vi "Untitled 1.vi"() -> ()   [LabVIEW 2020]
panel:
  in  "VISA resource name":refnum<visa-resource-name>
  in  "Table Control":string[][](table)
  out "Temp":dbl(graph)
  out "Thermometer":dbl(slide) scale=0.0..100.0
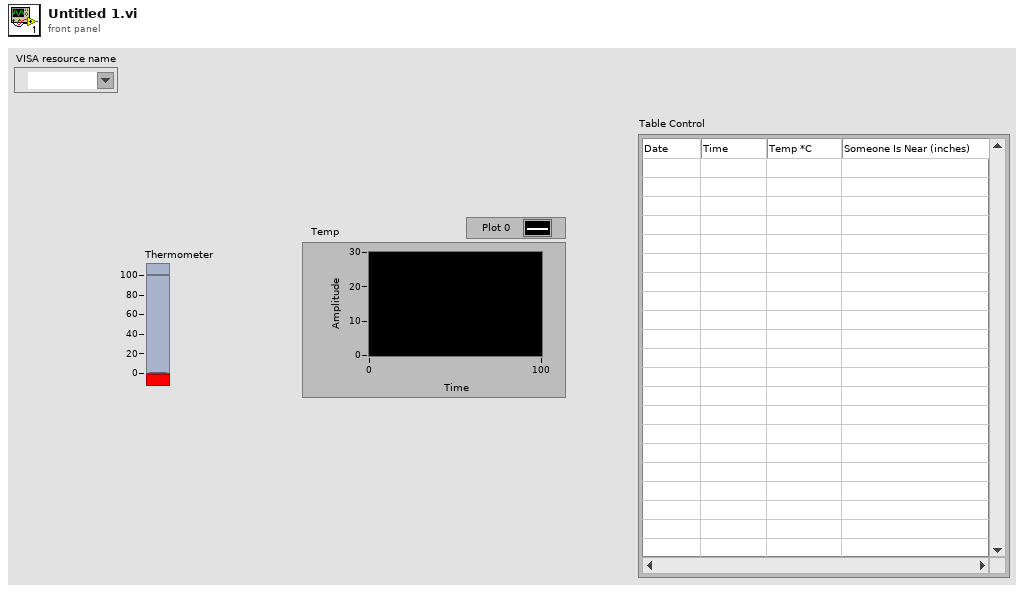
[diagram p1: front panel]
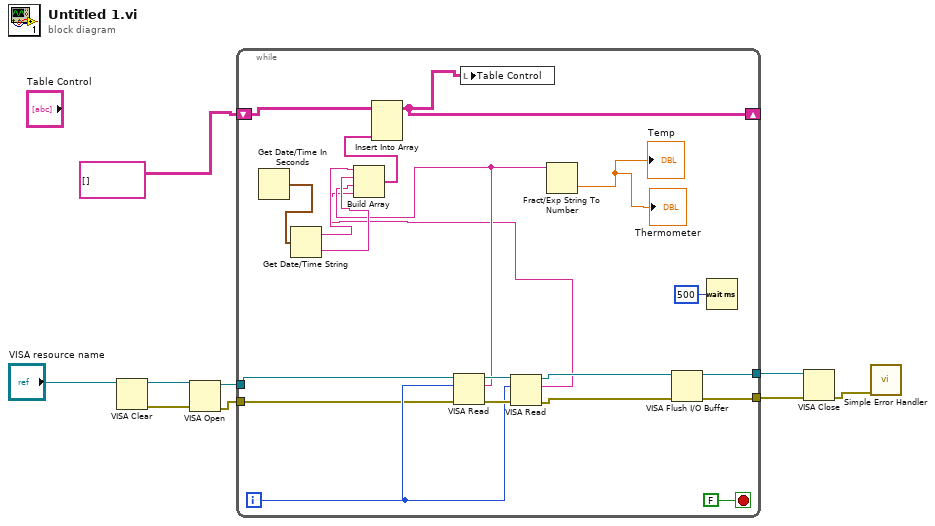
[diagram p0: block diagram]
diagram:
  n1 = VISA Clear(VISA resource name="VISA resource name") -> (VISA resource name out=w5:refnum<visa-resource-name>, error out=w6:errorcluster)  [unwired: 1 in]
  n2 = VISA Open(error in (no error)=w6, VISA resource name=w5) -> (VISA resource name=w4:refnum<visa-resource-name>, error out=w3:errorcluster)  [unwired: 3 in]
  n3 = while {
    tunnel: [w29] -> w8
    tunnel: [w28] -> w7
    tunnel: w4 -> [w22]
    tunnel: w3 -> [w21]
    shift-right: [w18] -> _
    shift-left: string[][] [] -> [w19]
    i -> [w23]
    stop <- FALSE stop-if-true
    n4 = Get Date/Time In Seconds() -> (seconds since 1Jan1904=w16:timestamp)
    n5 = Get Date/Time String(seconds (now)=w16) -> (date string=w15:string, time string=w14:string)  [unwired: 2 in]
    n6 = VISA Read(VISA resource name=w22, byte count=w23, error in (no error)=w21) -> (VISA resource name out=w25:refnum<visa-resource-name>, read buffer=w13:string, error out=w24:errorcluster)  [unwired: 1 out]
    n7 = VISA Read(VISA resource name=w25, byte count=w23, error in (no error)=w24) -> (VISA resource name out=w27:refnum<visa-resource-name>, read buffer=w11:string, error out=w26:errorcluster)  [unwired: 1 out]
    n8 = Build Array(w15, w14, w13, w11) -> (w10:string[])
    n9 = Insert Into Array(array=w19, new element=w10) -> (w18:string[][])  [unwired: 2 in]
    n10 = local write "Table Control"(w18) -> ()
    n11 = Fract/Exp String To Number(string=w13) -> (number=→"Thermometer" →"Temp":dbl)  [unwired: 3 in, 1 out]
    n12 = VISA Flush I/O Buffer(VISA resource name=w27, error in (no error)=w26) -> (VISA resource name out=w29:refnum<visa-resource-name>, error out=w28:errorcluster)  [unwired: 1 in]
    n13 = Wait (ms)(milliseconds to wait=u32 500) -> ()  [unwired: 1 out]
  }
  n14 = VISA Close(VISA resource name=w8, error in (no error)=w7) -> (error out=w9:errorcluster)
  n15 = call <vilib>:"Simple Error Handler.vi"("error in (no error)"=w9) -> ()  [unwired: 4 in, 5 out]
